vi "load array file.vi"(10 "2d?":bool, 11 "Data Form":T1) -> (3 "File Array Out":path[](array[path]))   [LabVIEW 2023]
uses:
  control/Data Form.ctl
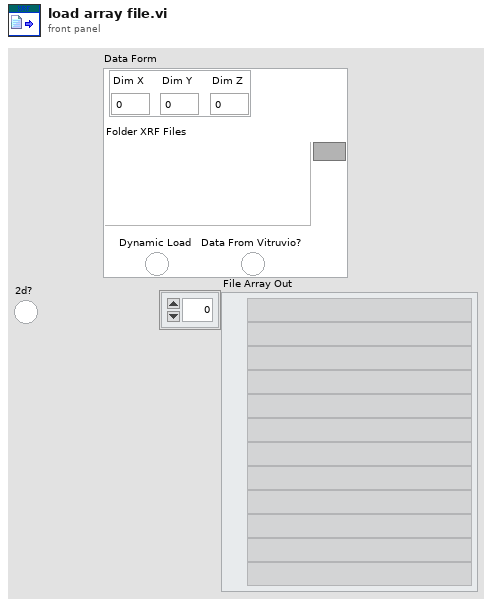
[diagram p1: front panel]
types:
  T1 = typedef "Data Form.ctl" = cluster{"Dimensions":cluster{"Dim X":i32, "Dim Y":i32, "Dim Z":i32}, "Folder XRF Files":path, "Dynamic Load":bool, "Data From Vitruvio?":bool}
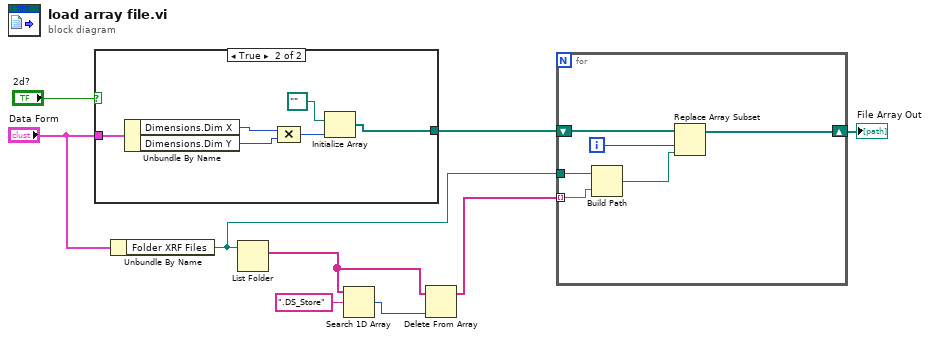
[diagram p0: block diagram]
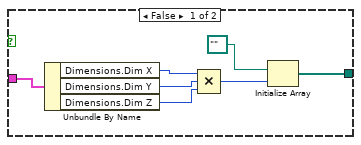
[diagram p2: hidden frame]
diagram:
  n1 = case shown="True" "2d?" {
    tunnel: "Data Form" -> [w13 w22]
    tunnel: [w10 w17] -> w7
    frame False {
      n2 = Unbundle By Name(w13) -> ("Dimensions.Dim X"=w16:i32, "Dimensions.Dim Y"=w15:i32, "Dimensions.Dim Z"=w12:i32)
      n3 = Compound Arithmetic op=MULTIPLY(w16, w15, w12) -> (w11:i32)
      n4 = Initialize Array(path "", w11) -> (w10:path[])
    }
    frame True {
      n5 = Unbundle By Name(w22) -> ("Dimensions.Dim X"=w21:i32, "Dimensions.Dim Y"=w20:i32)
      n6 = Compound Arithmetic op=MULTIPLY(w21, w20) -> (w19:i32)
      n7 = Initialize Array(path "", w19) -> (w17:path[])
    }
  }
  n8 = Unbundle By Name("Data Form") -> ("Folder XRF Files"=w2:path)
  n9 = List Folder(path=w2) -> (filenames=w4:string[])  [unwired: 3 in, 3 out]
  n10 = Search 1D Array(1D array=w4, element=".DS_Store") -> (index of element=w6:i32)  [unwired: 1 in]
  n11 = Delete From Array(array=w4, index=w6) -> (array with subset deleted=w3:string[])  [unwired: 1 in, 1 out]
  n12 = for {
    tunnel: w3 -> [w27] mode=indexing
    tunnel: w2 -> [w28]
    shift-right: [w23] -> w1
    shift-left: w7 -> [w26]
    i -> [w25]
    n13 = Build Path(base path=w28, name or relative path=w27) -> (appended path=w24:path)
    n14 = Replace Array Subset(array=w26, new element=w24, index=w25) -> (w23:path[])
  }
  "File Array Out" <- w1
